vi "Service Mode Version Parse HE.vi"(0 "GEA2 Reference In":refnum<k24>, 5 "Version Selection":T1, 11 "Error In":errorcluster) -> (3 "Non Crit Version 2":string, 4 "GEA2 Reference Out":refnum<k24>, 6 "Crit Version 1":string, 8 "Crit Version 2":string, 10 "Non Crit Version 1":string, 15 "Error Out":errorcluster)   [LabVIEW 2016, in "TLMB.lvlib"]
uses:
  Projects/TLMB.lvlib
  Q:/Common/DLLs/GEA3/GeaCommunication.dll
  Common/DLLs/GEA3/GeaCommunication.dll
  type defs/Service Mode Version Selection.ctl
  Common/LabVIEW GEA2 Toolkit/LabVIEW_GEA2_Toolkit.lvlibp/type defs/Source_Destination.ctl
  Common/LabVIEW GEA2 Toolkit/LabVIEW_GEA2_Toolkit.lvlibp/type defs/ERD Read Data In.ctl
  Common/LabVIEW GEA2 Toolkit/LabVIEW_GEA2_Toolkit.lvlibp/type defs/Data Type.ctl
  Common/LabVIEW GEA2 Toolkit/LabVIEW_GEA2_Toolkit.lvlibp
panel:
  in  "Standalone?":bool
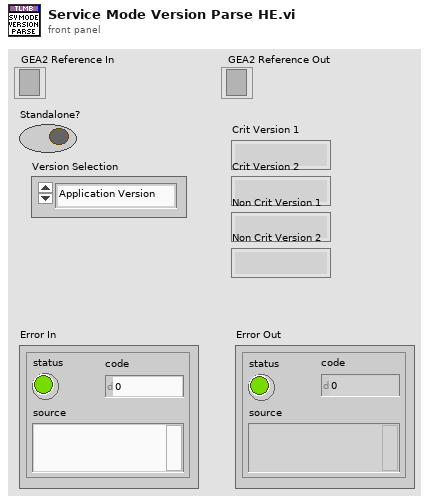
[diagram p1: front panel]
types:
  T1 = typedef "TLMB.lvlib/Service Mode Version Selection.ctl" = enum16{"Application Version", "XML Version"}
  T2 = typedef "LabVIEW_GEA2_Toolkit.lvlibp/Source_Destination.ctl" = cluster{"Source":u8, "Destination":u8}
  T3 = typedef "LabVIEW_GEA2_Toolkit.lvlibp/ERD Read Data In.ctl" = cluster{"ERD Number":u16, "Data Type":T4}
  T4 = typedef "LabVIEW_GEA2_Toolkit.lvlibp/Data Type.ctl" = enum16{"string", "boolean", "uint8_t", "uint16_t", "uint32_t", "uint64_t", "int8_t", "int16_t", "int32_t", "int64_t"}
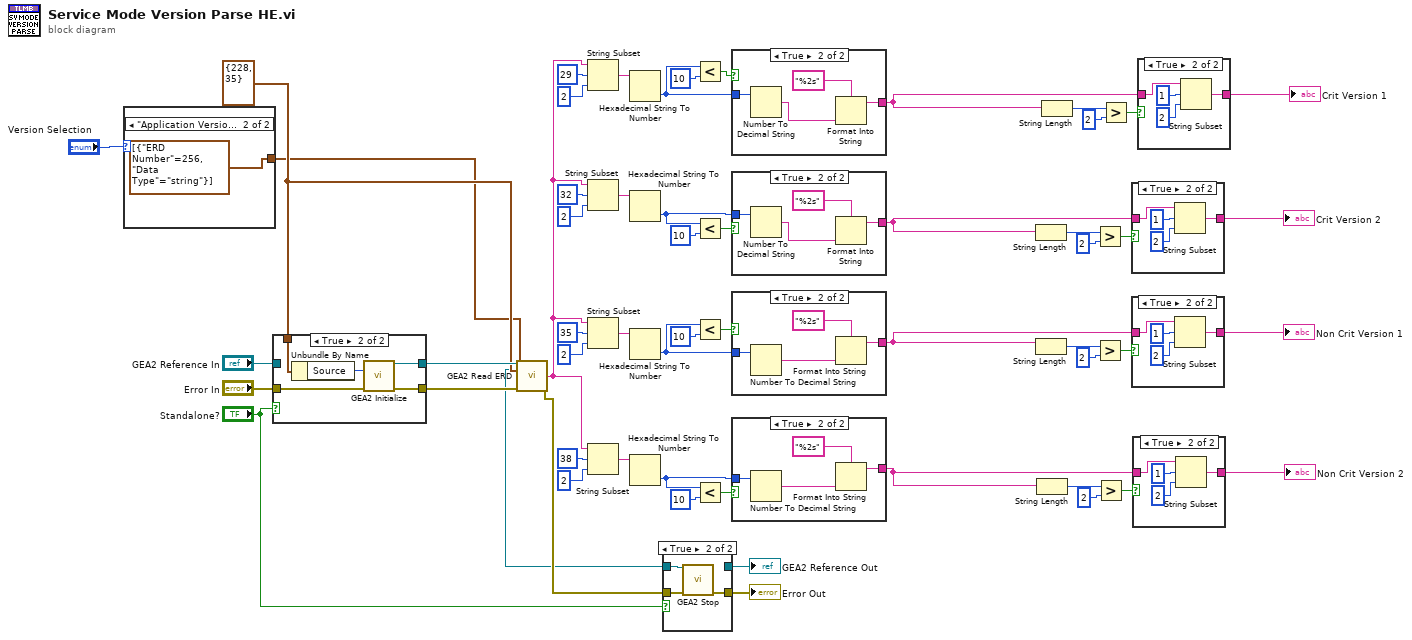
[diagram p0: block diagram]
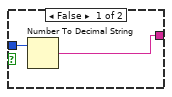
[diagram p6: hidden frame]
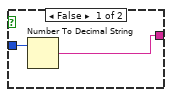
[diagram p7: hidden frame]
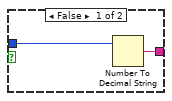
[diagram p8: hidden frame]
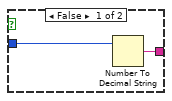
[diagram p9: hidden frame]
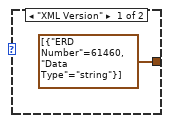
[diagram p10: hidden frame]
diagram:
  w49 = T2 {"Source"=228, "Destination"=35} ("GEA Inputs")
  n1 = case shown="\"Application Version\", Default" "Version Selection" {
    tunnel: [T3[] [{"ERD Number"=61460, "Data Type"=enum."string"}] ("Read ERD List") T3[] [{"ERD Number"=256, "Data Type"=enum."string"}] ("Read ERD List")] -> w47
    frame "XML Version" {
    }
    frame "Application Version", Default {
    }
  }
  n2 = case shown="True" "Standalone?" {
    tunnel: "Error In" -> [w60 w66]
    tunnel: [w60 w65] -> w52
    tunnel: "GEA2 Reference In" -> [w61 _]
    tunnel: [w61 w64] -> w50
    tunnel: w49 -> [_ w62]
    frame False {
    }
    frame True {
      n3 = Unbundle By Name(w62) -> ("Source"=w63:u8)
      n4 = call "GEA2 Initialize.vi"("Source Address"=w63, "error in"=w66) -> ("GEA2 Reference Out"=w64:refnum<k24>, "error out"=w65:errorcluster)  [unwired: 11 in, 1 out]
    }
  }
  n5 = call "GEA2 Read ERD.vi"("GEA2 Reference In"=w50, "GEA Inputs"=w49, "Read ERD List"=w47, "Error In"=w52) -> ("GEA2 Reference Out"=w48:refnum<k24>, "Raw Data Out"=w37:string, "Error Out"=w51:errorcluster)  [unwired: 8 in, 1 out]
  n6 = String Subset(string=w37, offset (0)=29, length (rest)=2 ("length (rest)")) -> (substring=w36:string)
  n7 = String Subset(string=w37, offset (0)=32, length (rest)=2 ("length (rest)")) -> (substring=w35:string)
  n8 = String Subset(string=w37, offset (0)=35, length (rest)=2 ("length (rest)")) -> (substring=w34:string)
  n9 = String Subset(string=w37, offset (0)=38, length (rest)=2 ("length (rest)")) -> (substring=w33:string)
  n10 = Hexadecimal String To Number(string=w36) -> (number=w32:u32)  [unwired: 2 in, 1 out]
  n11 = Hexadecimal String To Number(string=w35) -> (number=w27:u32)  [unwired: 2 in, 1 out]
  n12 = Hexadecimal String To Number(string=w34) -> (number=w24:u32)  [unwired: 2 in, 1 out]
  n13 = Hexadecimal String To Number(string=w33) -> (number=w21:u32)  [unwired: 2 in, 1 out]
  n14 = case shown="True" "Standalone?" {
    tunnel: [w67 w71] -> w55
    tunnel: w48 -> [w68 w70]
    tunnel: [w68 _] -> w54
    tunnel: w51 -> [w67 w69]
    frame False {
    }
    frame True {
      n15 = call "GEA2 Stop.vi"("GEA2 Reference In"=w70, "Error In"=w69) -> ("Error Out"=w71:errorcluster)  [unwired: 13 in]
    }
  }
  "Error Out" <- w55
  "GEA2 Reference Out" <- w54
  n16 = Less?(x=w32, y=u32 10) -> (x < y?=w30:bool)
  n17 = Less?(x=w27, y=u32 10) -> (x < y?=w28:bool)
  n18 = Less?(x=w24, y=u32 10) -> (x < y?=w25:bool)
  n19 = Less?(x=w21, y=u32 10) -> (x < y?=w22:bool)
  n20 = case shown="True" w30 {
    tunnel: [w72 w77] -> w20
    tunnel: w32 -> [w73 w74]
    frame False {
      n21 = Number To Decimal String(number=w73) -> (decimal integer string=w72:string)  [unwired: 1 in]
    }
    frame True {
      n22 = Number To Decimal String(number=w74) -> (decimal integer string=w76:string)  [unwired: 1 in]
      n23 = Format Into String(format string="%2s", w76) -> (resulting string=w77:string)  [unwired: 2 in, 1 out]
    }
  }
  n24 = case shown="True" w28 {
    tunnel: [w78 w83] -> w17
    tunnel: w27 -> [w79 w80]
    frame False {
      n25 = Number To Decimal String(number=w79) -> (decimal integer string=w78:string)  [unwired: 1 in]
    }
    frame True {
      n26 = Number To Decimal String(number=w80) -> (decimal integer string=w82:string)  [unwired: 1 in]
      n27 = Format Into String(format string="%2s", w82) -> (resulting string=w83:string)  [unwired: 2 in, 1 out]
    }
  }
  n28 = case shown="True" w25 {
    tunnel: [w84 w89] -> w18
    tunnel: w24 -> [w85 w86]
    frame False {
      n29 = Number To Decimal String(number=w85) -> (decimal integer string=w84:string)  [unwired: 1 in]
    }
    frame True {
      n30 = Number To Decimal String(number=w86) -> (decimal integer string=w88:string)  [unwired: 1 in]
      n31 = Format Into String(format string="%2s", w88) -> (resulting string=w89:string)  [unwired: 2 in, 1 out]
    }
  }
  n32 = case shown="True" w22 {
    tunnel: [w90 w95] -> w19
    tunnel: w21 -> [w91 w92]
    frame False {
      n33 = Number To Decimal String(number=w91) -> (decimal integer string=w90:string)  [unwired: 1 in]
    }
    frame True {
      n34 = Number To Decimal String(number=w92) -> (decimal integer string=w94:string)  [unwired: 1 in]
      n35 = Format Into String(format string="%2s", w94) -> (resulting string=w95:string)  [unwired: 2 in, 1 out]
    }
  }
  n36 = String Length(string=w17) -> (length=w10:i32)
  n37 = String Length(string=w18) -> (length=w7:i32)
  n38 = String Length(string=w19) -> (length=w16:i32)
  n39 = String Length(string=w20) -> (length=w13:i32)
  n40 = Greater?(x=w10, y=2) -> (0:w8:bool)
  n41 = Greater?(x=w7, y=2) -> (0:w5:bool)
  n42 = Greater?(x=w16, y=2) -> (0:w14:bool)
  n43 = Greater?(x=w13, y=2) -> (0:w11:bool)
  n44 = case shown="True" w8 {
    tunnel: [w96 w100] -> w3
    tunnel: w17 -> [w96 w97]
    frame False {
    }
    frame True {
      n45 = String Subset(string=w97, offset (0)=1, length (rest)=2 ("length (rest)")) -> (substring=w100:string)
    }
  }
  "Crit Version 2" <- w3
  n46 = case shown="True" w5 {
    tunnel: [w101 w105] -> w2
    tunnel: w18 -> [w101 w102]
    frame False {
    }
    frame True {
      n47 = String Subset(string=w102, offset (0)=1, length (rest)=2 ("length (rest)")) -> (substring=w105:string)
    }
  }
  "Non Crit Version 1" <- w2
  n48 = case shown="True" w14 {
    tunnel: [w106 w110] -> w1
    tunnel: w19 -> [w106 w107]
    frame False {
    }
    frame True {
      n49 = String Subset(string=w107, offset (0)=1, length (rest)=2 ("length (rest)")) -> (substring=w110:string)
    }
  }
  "Non Crit Version 2" <- w1
  n50 = case shown="True" w11 {
    tunnel: [w111 w115] -> w4
    tunnel: w20 -> [w111 w112]
    frame False {
    }
    frame True {
      n51 = String Subset(string=w112, offset (0)=1, length (rest)=2 ("length (rest)")) -> (substring=w115:string)
    }
  }
  "Crit Version 1" <- w4
